vi "Convert Signal.vi"(0 "Pressure":dbl[](array[numeric]), 1 "error in (no error)":errorcluster) -> (2 "Array":dbl[](array[numeric]), 3 "df":dbl, 4 "error out":errorcluster)   [LabVIEW 2017]
uses:
  <vilib>/measure/maspectr.llb/FFT Spectrum (Mag-Phase) for 1 Chan.vi
  <vilib>/measure/NI_MAPro.lvlib
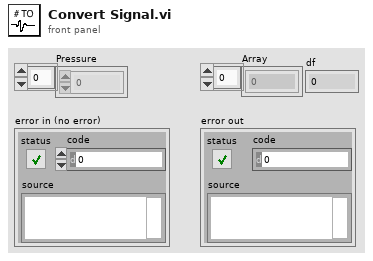
[diagram p1: front panel]
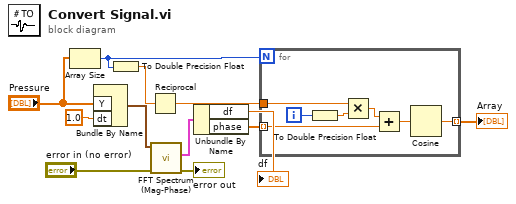
[diagram p0: block diagram]
diagram:
  n1 = Array Size(array="Pressure") -> (size(s)=w7:i32)
  n2 = Bundle By Name("Y"="Pressure", "dt"=1.0) -> (w3:waveform(dbl))  [unwired: 1 in]
  n3 = To Double Precision Float(number=w7) -> (double precision float=w6:dbl)
  n4 = Reciprocal(x=w6) -> (1/x=w8:dbl)
  n5 = call-poly <vilib>:"FFT Spectrum (Mag-Phase).vi"("error in (no error)"="error in (no error)", "time signal"=w3) -> ("error out"=→"error out":errorcluster, "phase"=w10:cluster{"f0":dbl, "df":dbl, "phase":dbl[]})  [unwired: 5 in, 3 out]
  n6 = Unbundle By Name(w10) -> ("df"=→"df":dbl, "phase"=w11:dbl[])
  n7 = for {
    N: w7 -> [_]
    tunnel: w8 -> [w19]
    tunnel: w11 -> [w15] mode=indexing
    tunnel: [w13] -> w9 mode=indexing
    i -> [w18]
    n8 = To Double Precision Float(number=w18) -> (double precision float=w17:dbl)
    n9 = Multiply(x=w19, y=w17) -> (x*y=w16:dbl)
    n10 = Add(x=w16, y=w15) -> (x+y=w14:dbl)
    n11 = Cosine(x=w14) -> (cos(x)=w13:dbl)
  }
  "Array" <- w9
